vi "Event-Driven State Machine.vi"() -> ()   [LabVIEW 2020]
uses:
  support/State Machine Data.ctl
  support/States.ctl
  <vilib>/DAQmx/read.llb/DAQmx Read (Analog 2D DBL NChan NSamp).vi
  <vilib>/DAQmx/write.llb/DAQmx Write (Analog DBL 1Chan 1Samp).vi
  <vilib>/DAQmx/create/channels.llb/DAQmx Create Channel (AI-Voltage-Basic).vi
  <vilib>/DAQmx/configure/timing.llb/DAQmx Timing (Sample Clock).vi
  <vilib>/DAQmx/miscellaneous.llb/DAQmx Fill In Error Info.vi
  <vilib>/Utility/file.llb/Write Delimited Spreadsheet (DBL).vi
  <vilib>/DAQmx/create/channels.llb/DAQmx Create Channel (AO-Voltage-Basic).vi
panel:
  out "RMS Results Per Channel":dbl[](array[numeric])
  out "Threshold exceeded?":bool
  in  "Acquire":bool
  in  "Samples per channel":i32=100
  in  "Sample Rate":dbl=1000.0
  in  "AI Voltage Channel":tag="PCI-6221/ai0, PCI-6221/ai2:3"
  in  "AO Voltage Channel":tag="PCI-6221/ao0"
  in  "Generate Stimulus":bool
  in  "Threshold (rms)":dbl=1.0
  in  "Clear":bool
  in  "Exit":bool
  out "Graph":dbl[][](graph)
  # "Analysis"
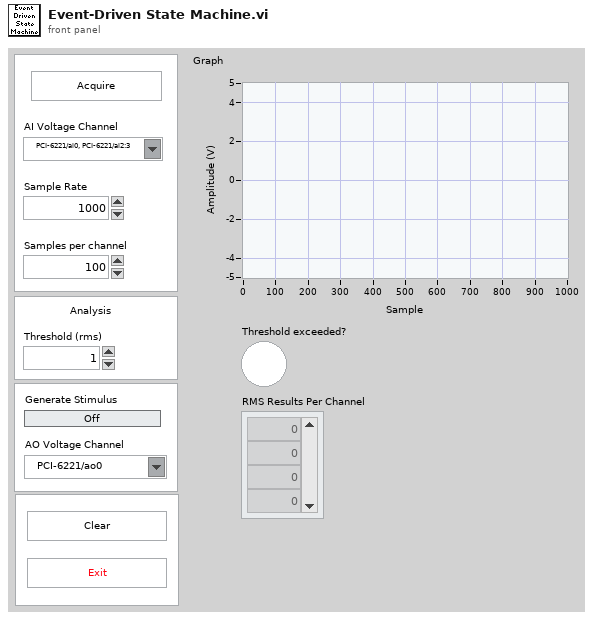
[diagram p1: front panel]
types:
  T1 = typedef "States.ctl" = enum16{"Initialize", "Wait for Event", "Acquire", "Analyze", "Log", "Clear", "Update Stimulus", "Update Graph", "Exit"}
  T2 = typedef "State Machine Data.ctl" = cluster{"Acquisition Data":dbl[][], "Stimulus Value":bool, "AO Voltage Channel":tag}
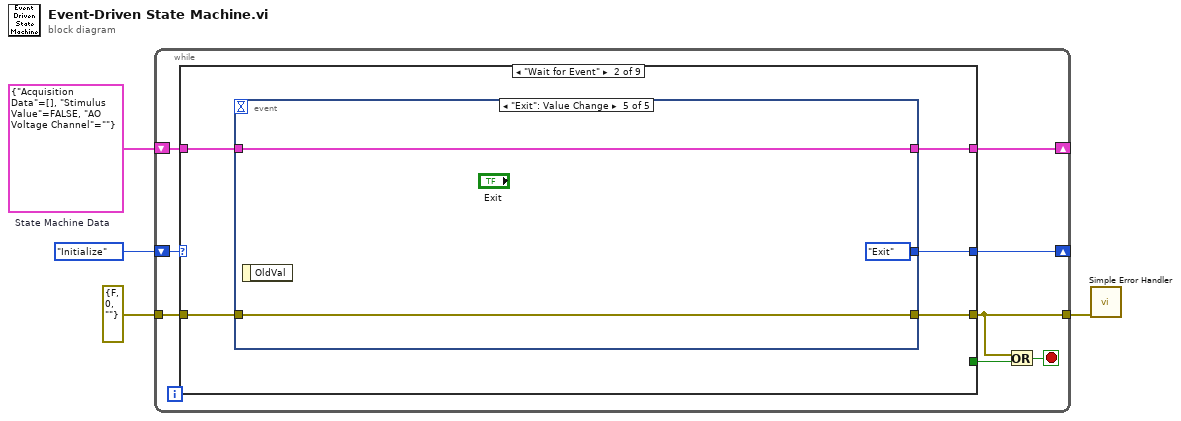
[diagram p0: block diagram]
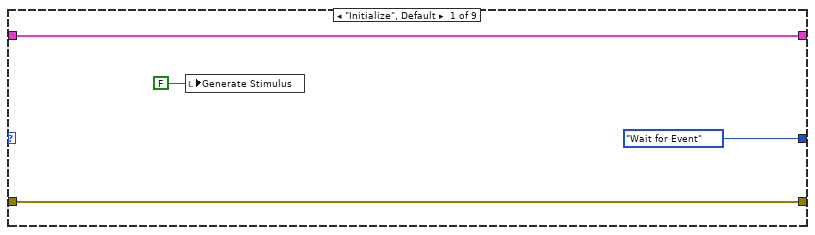
[diagram p2: hidden frame]
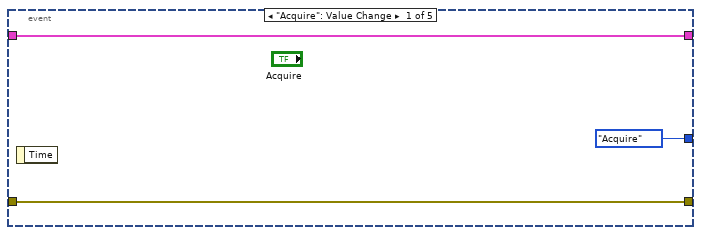
[diagram p3: hidden frame]
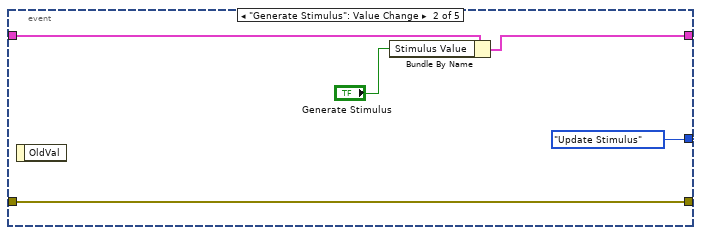
[diagram p4: hidden frame]
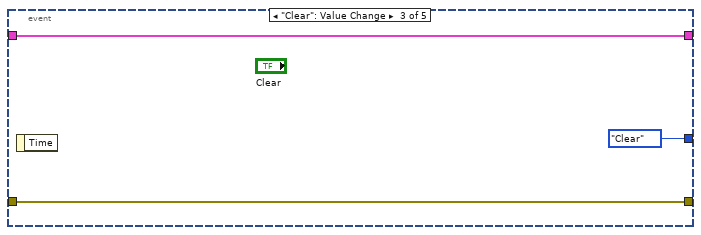
[diagram p5: hidden frame]
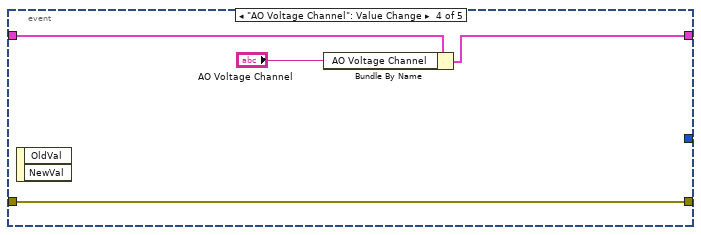
[diagram p6: hidden frame]
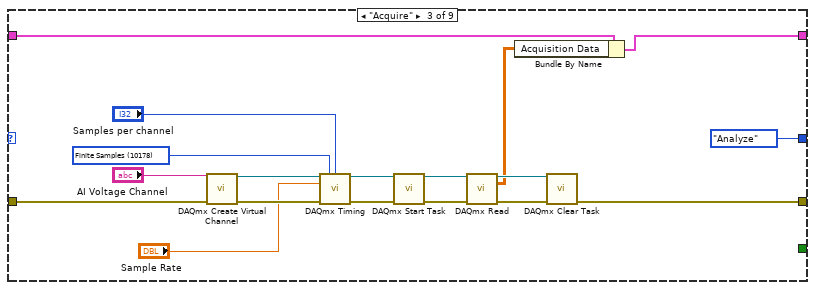
[diagram p7: hidden frame]
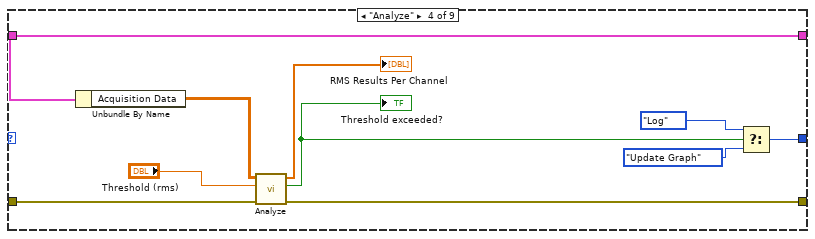
[diagram p8: hidden frame]
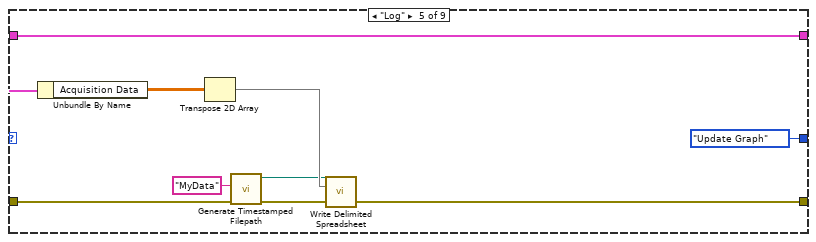
[diagram p9: hidden frame]
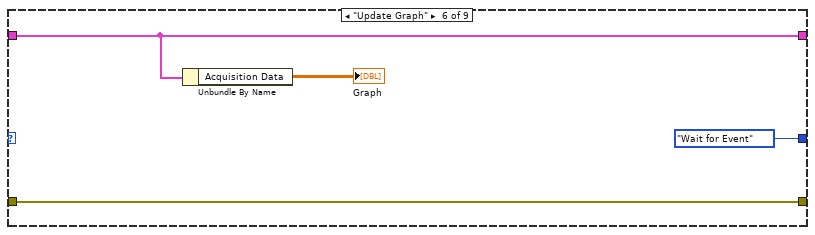
[diagram p10: hidden frame]
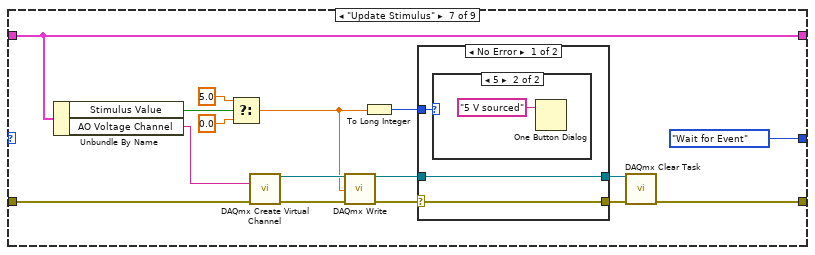
[diagram p11: hidden frame]
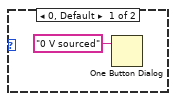
[diagram p12: hidden frame]
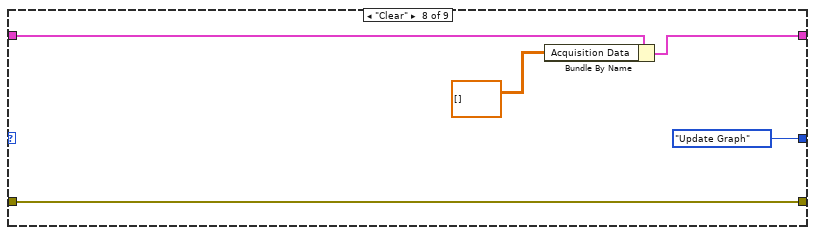
[diagram p14: hidden frame]
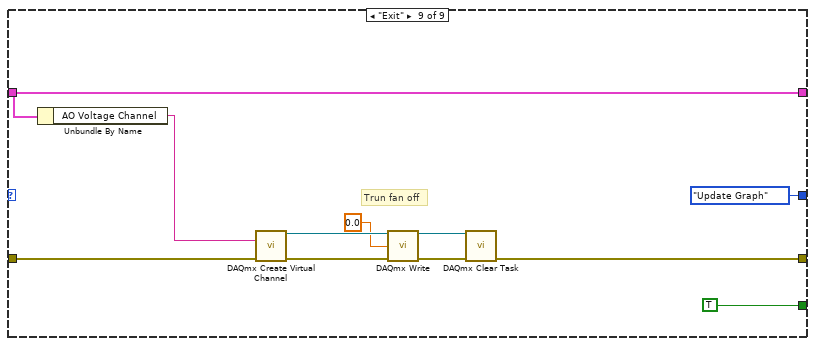
[diagram p15: hidden frame]
diagram:
  w3 = T2 {"Acquisition Data"=[], "Stimulus Value"=FALSE, "AO Voltage Channel"=""}  # State Machine Data
  n1 = while {
    shift-right: [w9] -> _
    shift-left: States."Initialize" ("States") -> [w12]
    shift-right: [w10] -> _
    shift-left: w3 -> [w11]
    tunnel: errorcluster {"status"=FALSE, "code"=0, "source"=""} ("error constant") -> [w8]
    tunnel: [w7] -> w1
    stop <- w5 stop-if-true
    n2 = case shown="\"Wait for Event\"" w12 {
      tunnel: w11 -> [w14 w21 w45 w67 w75 w79 w96 w107 w110]
      tunnel: [w14 w20 w41 w67 w75 w79 w96 w105 w110] -> w10
      tunnel: [States."Wait for Event" ("States") w17 States."Analyze" ("States") w59 States."Update Graph" ("States") States."Wait for Event" ("States") States."Wait for Event" ("States") States."Update Graph" ("States") States."Update Graph" ("States")] -> w9
      tunnel: w8 -> [w15 w19 w57 w64 w73 w80 w90 w108 w113]
      tunnel: [w15 w18 w43 w62 w69 w80 w91 w108 w112] -> w7
      tunnel: [_ _ _ _ _ _ _ _ TRUE] -> w6
      frame "Initialize", Default {
        n3 = local write "Generate Stimulus"(FALSE ("Stimulus Value")) -> ()
      }
      frame "Wait for Event" {
        n4 = event shown="[4] \"Exit\": Value Change" {
          selector: _ -> [_ _ _ _ _]
          dyn-events: _ -> [_ _ _ _ _]
          timeout: _ -> [_ _ _ _ _]
          tunnel: w21 -> [w23 w29 w32 w36 w38]
          tunnel: [w23 w28 w32 w34 w38] -> w20
          tunnel: w19 -> [w24 w27 w31 w33 w39]
          tunnel: [w24 w27 w31 w33 w39] -> w18
          tunnel: [States."Acquire" ("Enum") States."Update Stimulus" ("Enum") States."Clear" ("Enum") _ States."Exit" ("Enum")] -> w17
          event "Acquire": Value Change {
            n5 = event-data() -> ()  [unwired: 1 in, 1 out]
          }
          event "Generate Stimulus": Value Change {
            n6 = event-data() -> ()  [unwired: 1 in, 1 out]
            n7 = Bundle By Name(cluster=w29, "Stimulus Value"="Generate Stimulus") -> (w28:T2)
          }
          event "Clear": Value Change {
            n8 = event-data() -> ()  [unwired: 1 in, 1 out]
          }
          event "AO Voltage Channel": Value Change {
            n9 = event-data() -> ()  [unwired: 1 in, 2 out]
            n10 = Bundle By Name(cluster=w36, "AO Voltage Channel"="AO Voltage Channel") -> (w34:T2)
          }
          event "Exit": Value Change {
            n11 = event-data() -> ()  [unwired: 1 in, 1 out]
          }
        }
      }
      frame "Acquire" {
        w53 = 10178 items=["Finite Samples"=10178, "Continuous Samples"=10123, "Hardware Timed Single Point"=12522] ("sample mode")
        n12 = call-poly <vilib>:"DAQmx Create Virtual Channel.vi"("physical channels"="AI Voltage Channel", "error in"=w57) -> ("task out"=w54:refnum<k21>, "error out"=w55:errorcluster)  [unwired: 12 in]
        n13 = call-poly <vilib>:"DAQmx Timing.vi"("task/channels in"=w54, "sample mode"=w53, "samples per channel"="Samples per channel", "rate"="Sample Rate", "error in"=w55) -> ("task out"=w51:refnum<k21>, "error out"=w50:errorcluster)  [unwired: 9 in]
        n14 = call <vilib>:"DAQmx Start Task.vi"("task/channels in"=w51, "error in"=w50) -> ("task out"=w49:refnum<k21>, "error out"=w48:errorcluster)  [unwired: 12 in]
        n15 = call-poly <vilib>:"DAQmx Read.vi"("task/channels in"=w49, "error in"=w48) -> ("task out"=w47:refnum<k21>, "data"=w44:dbl[][], "error out"=w46:errorcluster)  [unwired: 11 in]
        n16 = Bundle By Name(cluster=w45, "Acquisition Data"=w44) -> (w41:T2)
        n17 = call <vilib>:"DAQmx Clear Task.vi"("task in"=w47, "error in"=w46) -> ("error out"=w43:errorcluster)  [unwired: 13 in]
      }
      frame "Analyze" {
        n18 = Unbundle By Name(w67) -> ("Acquisition Data"=w66:dbl[][])
        n19 = call "Analyze.vi"("error in (no error)"=w64, "Threshold (rms)"="Threshold (rms)", "N-Channel Data (2D DBL)"=w66) -> ("error out"=w62:errorcluster, "Threshold Exceeded?"=w58:bool, "N-Channel RMS Results"=→"RMS Results Per Channel":dbl[])  [unwired: 5 in, 1 out]
        "Threshold exceeded?" <- w58
        n20 = Select(t=States."Log" ("States"), s=w58, f=States."Update Graph" ("States")) -> (s? t:f=w59:T1)
      }
      frame "Log" {
        n21 = Unbundle By Name(w75) -> ("Acquisition Data"=w76:dbl[][])
        n22 = Transpose 2D Array(2D array=w76) -> (transposed array=w72:dbl[][])
        n23 = call "Generate Timestamped Filepath.vi"("Error In"=w73, "appended filename"="MyData") -> ("Error Out"=w70:errorcluster, "timestamped relative filepath"=w71:path)  [unwired: 8 in]
        n24 = call-poly <vilib>:"Write Delimited Spreadsheet.vi"("file path (dialog if empty)"=w71, "2D data"=w72, "error in (no error)"=w70) -> ("error out"=w69:errorcluster)  [unwired: 11 in, 1 out]
      }
      frame "Update Graph" {
        n25 = Unbundle By Name(w79) -> ("Acquisition Data"=→"Graph":dbl[][])
      }
      frame "Update Stimulus" {
        n26 = Unbundle By Name(w96) -> ("Stimulus Value"=w88:bool, "AO Voltage Channel"=w87:tag)
        n27 = Select(t=5.0, s=w88, f=0.0) -> (s? t:f=w86:dbl)
        n28 = call-poly <vilib>:"DAQmx Create Virtual Channel.vi"("physical channels"=w87, "error in"=w90) -> ("task out"=w93:refnum<k21>, "error out"=w92:errorcluster)  [unwired: 12 in]
        n29 = call-poly <vilib>:"DAQmx Write.vi"("task/channels in"=w93, "data"=w86, "error in"=w92) -> ("task out"=w82:refnum<k21>, "error out"=w84:errorcluster)  [unwired: 10 in, 1 out]
        n30 = To Long Integer(number=w86) -> (32bit integer=w85:i32)
        n31 = case shown="No Error" w84 {
          selector: w84 -> [w98 w102]
          tunnel: w85 -> [w99 _]
          tunnel: [w98 w102] -> w83
          tunnel: w82 -> [w97 w103]
          tunnel: [w97 w103] -> w81
          frame No Error {
            n32 = case shown="5" w99 {
              frame 0, Default {
                n33 = One Button Dialog(message="0 V sourced") -> ()  [unwired: 1 in, 1 out]
              }
              frame 5 {
                n34 = One Button Dialog(message="5 V sourced") -> ()  [unwired: 1 in, 1 out]
              }
            }
          }
          frame Error {
          }
        }
        n35 = call <vilib>:"DAQmx Clear Task.vi"("task in"=w81, "error in"=w83) -> ("error out"=w91:errorcluster)  [unwired: 13 in]
      }
      frame "Clear" {
        n36 = Bundle By Name(cluster=w107, "Acquisition Data"=dbl[][] []) -> (w105:T2)
      }
      frame "Exit" {
        # "Trun fan off"
        n37 = Unbundle By Name(w110) -> ("AO Voltage Channel"=w109:tag)
        n38 = call-poly <vilib>:"DAQmx Create Virtual Channel.vi"("physical channels"=w109, "error in"=w113) -> ("task out"=w114:refnum<k21>, "error out"=w115:errorcluster)  [unwired: 12 in]
        n39 = call-poly <vilib>:"DAQmx Write.vi"("task/channels in"=w114, "data"=0.0, "error in"=w115) -> ("task out"=w116:refnum<k21>, "error out"=w117:errorcluster)  [unwired: 10 in, 1 out]
        n40 = call <vilib>:"DAQmx Clear Task.vi"("task in"=w116, "error in"=w117) -> ("error out"=w112:errorcluster)  [unwired: 13 in]
      }
    }
    n41 = Or(x=w7, y=w6) -> (x .or. y?=w5:bool)
  }
  n42 = call <vilib>:"Simple Error Handler.vi"("error in (no error)"=w1) -> ()  [unwired: 4 in, 5 out]
